vi "Log Filenames List.vi"(8 "error in (no error)":errorcluster, 9 "Archive File Type":T1, 10 "LogFile Type":T2, 11 "Log Filename Actions":T3) -> (0 "error out":errorcluster, 2 "New File":bool, 3 "Filename":path)   [LabVIEW 2009]
uses:
  Log Filename Actions.ctl
  LogFileType.ctl
  Archive File Type.ctl
  Apps/App Parameters Actions.ctl
panel:
  out "Array":path[](array[path])
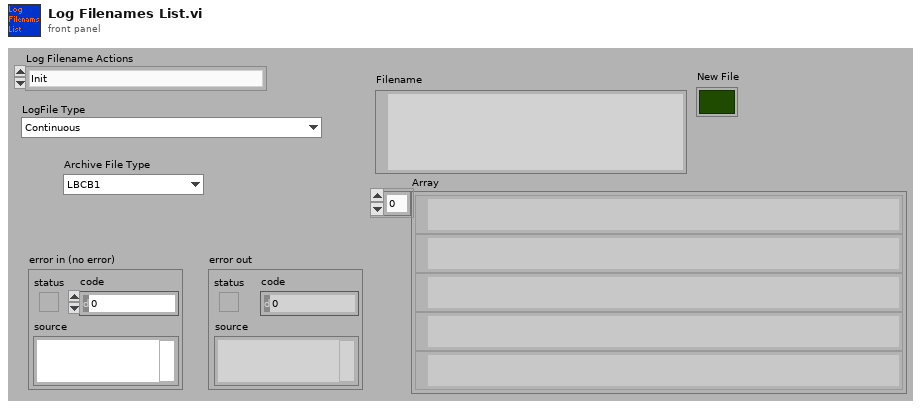
[diagram p1: front panel]
types:
  T1 = typedef "Archive File Type.ctl" = enum16{"LBCB1", "LBCB2", "ExternalSensors", "Combined"}
  T2 = typedef "LogFileType.ctl" = enum16{"Continuous", "Step", "Volts", "Offsets", "DLL  Errors", "Snapshot", "Commands", "StiffnessUpdates", "End List"}
  T3 = typedef "Log Filename Actions.ctl" = enum16{"Init", "Get Filename", "New Log Directory"}
  T4 = typedef "App Parameters Actions.ctl" = enum16{"Init", "Get", "Set"}
  T5 = typedef "App Parameters.ctl" = cluster{"Monitor Loop":T6, "Ramp Time":T6, "Log Loop":T6, "TCP to DAQ":T6, "Logging Directory":path, "Log File Size (MBytes)":i64, "Volt Logging Loop":T6, "2 LBCB Archiving Mode":bool}
  T6 = typedef "Timing Parameters.ctl" = cluster{"Interval":dbl, "Rate ":dbl}
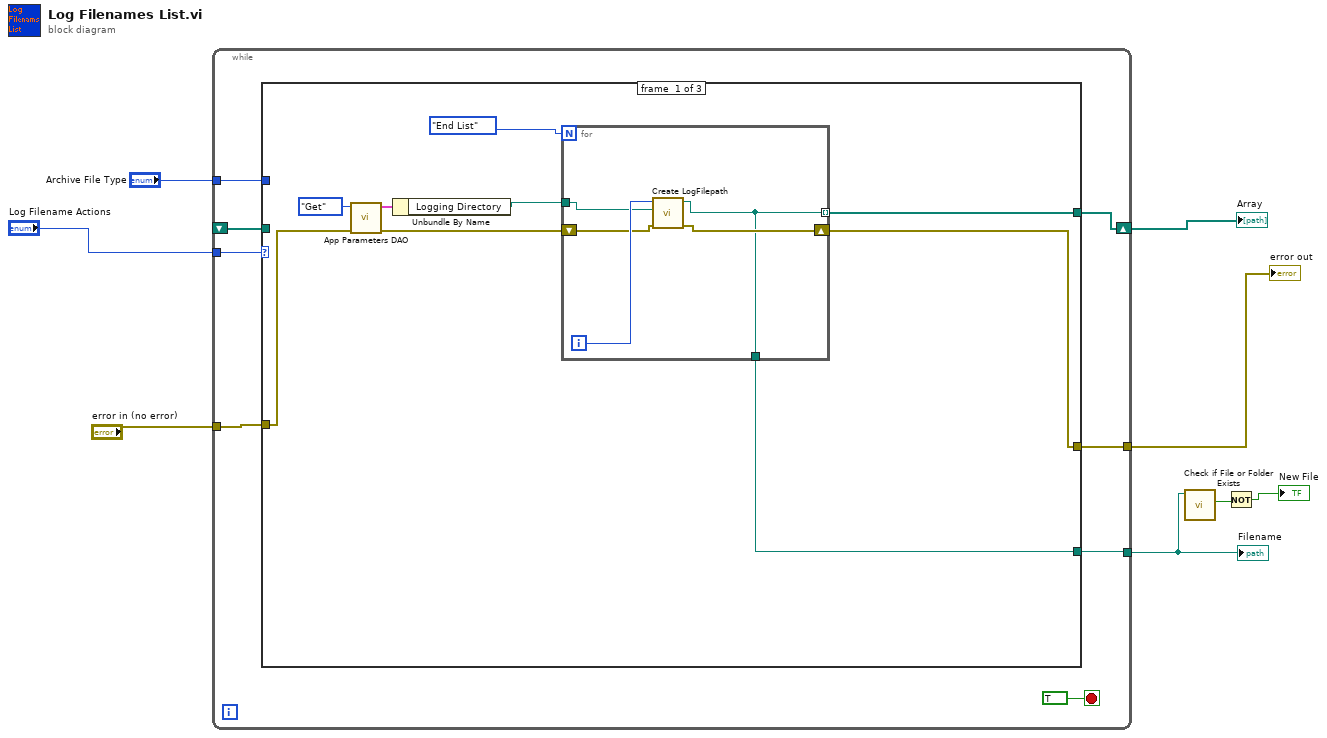
[diagram p0: block diagram]
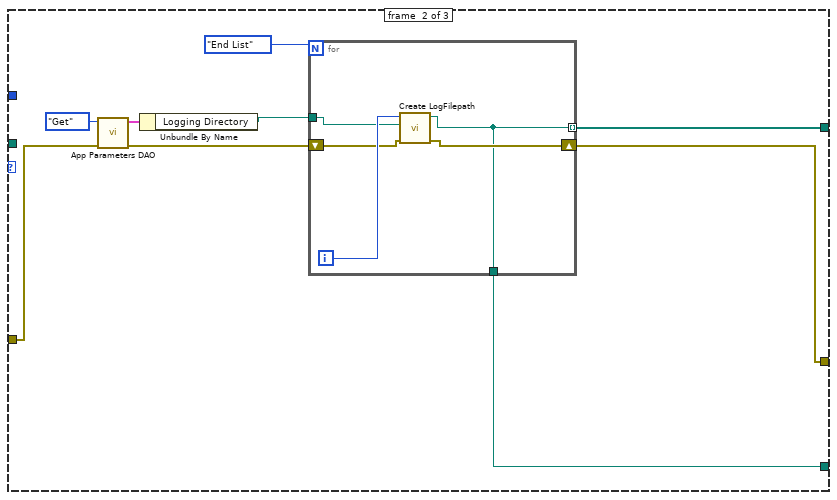
[diagram p2: hidden frame]
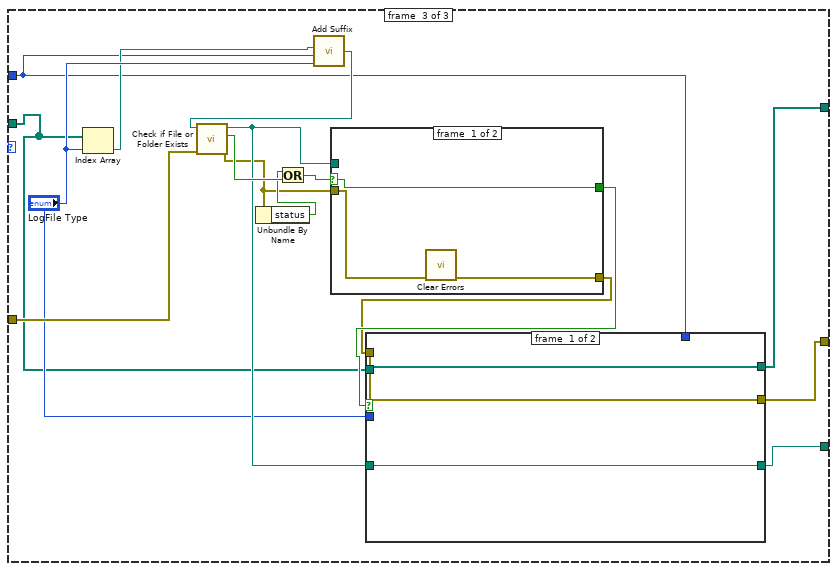
[diagram p3: hidden frame]
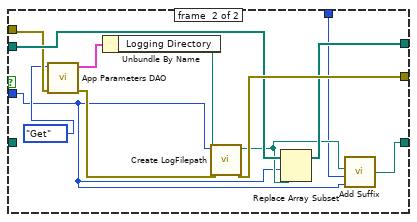
[diagram p4: hidden frame]
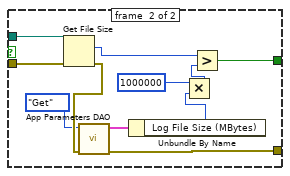
[diagram p5: hidden frame]
diagram:
  n1 = while {
    tunnel: "Log Filename Actions" -> [w15]
    shift-right: [w13] -> w5
    shift-left: _ -> [w14]
    tunnel: [w12] -> w3
    tunnel: "error in (no error)" -> [w11]
    tunnel: [w10] -> w6
    tunnel: "Archive File Type" -> [w9]
    stop <- TRUE stop-if-true
    n2 = case shown="\"Get Filename\"" w15 {
      tunnel: w14 -> [_ _ w48]
      tunnel: [w19 w32 w55] -> w13
      tunnel: [w17 w31 w54] -> w12
      tunnel: w11 -> [w24 w37 w60]
      tunnel: [w20 w33 w56] -> w10
      tunnel: w9 -> [_ _ w45]
      frame #0 {
        n3 = call "App Parameters DAO.vi"("error in (no error)"=w24, "Actions"=App_Parameters_Actions."Get" ("App Parameter Actions")) -> ("error out"=w21:errorcluster, "Application Timing and Logging Out"=w23:T5)  [unwired: 2 in, 6 out]
        n4 = Unbundle By Name(w23) -> ("Logging Directory"=w22:path)
        n5 = for {
          N: LogFileType."End List" ("LogFile Type") -> [_]
          tunnel: w22 -> [w29]
          shift-right: [w27] -> w20
          shift-left: w21 -> [w28]
          tunnel: [w26] -> w19 mode=indexing
          tunnel: [w26] -> w17
          i -> [w30]
          n6 = call "Create LogFilepath.vi"("error in (no error)"=w28, "Log Directory"=w29, "LogFile Type"=w30) -> ("error out"=w27:errorcluster, "Logfile Path"=w26:path)  [unwired: 7 out]
        }
      }
      frame #1 {
        n7 = call "App Parameters DAO.vi"("error in (no error)"=w37, "Actions"=App_Parameters_Actions."Get" ("App Parameter Actions")) -> ("error out"=w34:errorcluster, "Application Timing and Logging Out"=w36:T5)  [unwired: 2 in, 6 out]
        n8 = Unbundle By Name(w36) -> ("Logging Directory"=w35:path)
        n9 = for {
          N: LogFileType."End List" ("LogFile Type") -> [_]
          tunnel: w35 -> [w43]
          shift-right: [w41] -> w33
          shift-left: w34 -> [w42]
          tunnel: [w40] -> w32 mode=indexing
          tunnel: [w40] -> w31
          i -> [w44]
          n10 = call "Create LogFilepath.vi"("error in (no error)"=w42, "Log Directory"=w43, "LogFile Type"=w44) -> ("error out"=w41:errorcluster, "Logfile Path"=w40:path)  [unwired: 7 out]
        }
      }
      frame #2 {
        n11 = Index Array(array=w48, index="LogFile Type") -> (element=w47:path)
        n12 = call "Add Suffix.vi"("LogFile Type"="LogFile Type", "Archive File Type"=w45, "Logfile Path"=w47) -> ("appended path"=w46:path)  [unwired: 1 in]
        n13 = call <vilib>:"Check if File or Folder Exists.vi"("error in (no error)"=w60, "path"=w46) -> ("error out"=w50:errorcluster, "file or folder exists?"=w59:bool, "dup path"=w53:path)  [unwired: 7 out]
        n14 = Unbundle By Name(w50) -> ("status"=w51:bool)
        n15 = Or(x=w51, y=w59) -> (x .or. y?=w52:bool)
        n16 = case shown="True" w52 {
          selector: w52 -> [w78 _]
          tunnel: w53 -> [_ w89]
          tunnel: w50 -> [w77 w88]
          tunnel: [w78 w82] -> w58
          tunnel: [w76 w81] -> w57
          frame #0 {
            n17 = call <vilib>:"Clear Errors.vi"("error in (no error)"=w77) -> ("error out"=w76:errorcluster)  [unwired: 6 out]
          }
          frame #1 {
            n18 = Get File Size(file=w89, error in=w88) -> (size (in bytes)=w83:i64, 0:w87:errorcluster)  [unwired: 1 out]
            n19 = call "App Parameters DAO.vi"("error in (no error)"=w87, "Actions"=App_Parameters_Actions."Get" ("App Parameter Actions")) -> ("error out"=w81:errorcluster, "Application Timing and Logging Out"=w85:T5)  [unwired: 2 in, 6 out]
            n20 = Unbundle By Name(w85) -> ("Log File Size (MBytes)"=w84:i64)
            n21 = Multiply(x=1000000, y=w84) -> (x*y=w80:i64)
            n22 = Greater?(x=w83, y=w80) -> (0:w82:bool)
          }
        }
        n23 = case shown="True" w58 {
          tunnel: "LogFile Type" -> [_ w65]
          tunnel: w57 -> [w62 w70]
          tunnel: [w62 w73] -> w56
          tunnel: w48 -> [w63 w72]
          tunnel: [w63 w71] -> w55
          tunnel: [w61 w66] -> w54
          tunnel: w53 -> [w61 _]
          tunnel: w45 -> [_ w64]
          frame #0 {
          }
          frame #1 {
            n24 = call "App Parameters DAO.vi"("error in (no error)"=w70, "Actions"=App_Parameters_Actions."Get" ("App Parameter Actions")) -> ("error out"=w68:errorcluster, "Application Timing and Logging Out"=w75:T5)  [unwired: 2 in, 6 out]
            n25 = Unbundle By Name(w75) -> ("Logging Directory"=w74:path)
            n26 = call "Create LogFilepath.vi"("error in (no error)"=w68, "Log Directory"=w74, "LogFile Type"=w65) -> ("error out"=w73:errorcluster, "Logfile Path"=w67:path)  [unwired: 7 out]
            n27 = Replace Array Subset(array=w72, new element=w67, index=w65) -> (w71:path[])
            n28 = call "Add Suffix.vi"("LogFile Type"=w65, "Archive File Type"=w64, "Logfile Path"=w67) -> ("appended path"=w66:path)  [unwired: 1 out]
          }
        }
      }
    }
  }
  "error out" <- w6
  "Filename" <- w3
  "Array" <- w5
  n29 = call <vilib>:"Check if File or Folder Exists.vi"("path"=w3) -> ("file or folder exists?"=w2:bool)  [unwired: 1 in, 9 out]
  n30 = Not(x=w2) -> (.not. x?=→"New File":bool)
